vi "Input Registers Engine.vi"(10 "Parameters":variant, 11 "Process":refnum<class "Process.lvclass">) -> ()   [LabVIEW 2021, in "FPGA Addon Engine.lvlib"]
uses:
  FPGA Addon Engine.lvlib
  <vilib>/NI/NIVS Inline Async API/_VS Inline Async API/Process/Process.lvclass
  Types/Register Settings.ctl
  Addon Shared/Types/FPGA Addon Data Type.ctl
  Addon Shared/Types/Scalar Type.ctl
  <vilib>/NI/NIVS Inline Async API/_VS Inline Async API/Process/Process.lvclass/Process.ctl
  <vilib>/Platform/TimedLoop/XDataNode/timing_clust.ctl
  <vilib>/Platform/TimedLoop/XDataNode/nitl_modes.ctl
  <vilib>/Platform/TimedLoop/XDataNode/wakeup.ctl
  <vilib>/NI/NIVS Inline Async API/_Data Access Engine/Access Type Classes/Write/Write.lvclass/Write.ctl
  <vilib>/NI/NIVS Inline Async API/_Data Access Engine/Data Access Engine/Methods/Write.Data.vi
  <vilib>/NI/NIVS Inline Async API/_VS Inline Async API/Process/Data Member Access/Read Data Access.vi
  <vilib>/NI/NIVS Inline Async API/_VS Inline Async API/Error Handling Process/SubVIs/Error.ConvertArray.vi
  <vilib>/NI/NIVS Inline Async API/_Data Access Engine/Access Type Classes/Write/Write.ProcessData.vi
  <vilib>/NI/NIVS Inline Async API/_Data Access Engine/Access Type Classes/Write/Write.Buffer.vi
  <vilib>/NI/NIVS Inline Async API/_Data Access Engine/Access Type Classes/Write/Write.Commit.vi
  Addon Shared/SubVIs/Constants.vi
  <vilib>/NI/NIVS Inline Async API/_Data Access Engine/Data Access Engine/Methods/Write.Lookup.vi
  <vilib>/NI/NIVS Inline Async API/_Data Access Engine/Data Access Engine/Data Access Engine.lvclass
  <vilib>/platform/TimedLoop/XDataNode/XDataNode.xnode
  Addon Shared/FPGA Addon Shared.lvlib
  <vilib>/Platform/TimedLoop/XDataNode/XDNodeRunTimeDep.lvlib
panel:
  out "error out":errorcluster
  in  "error in (no error)":errorcluster
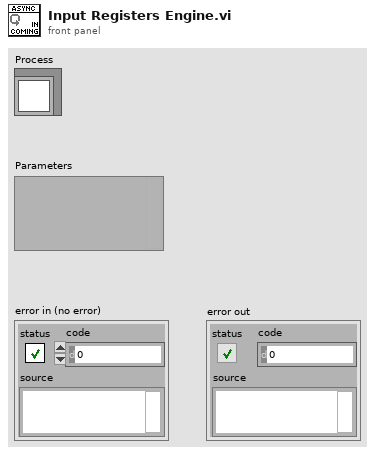
[diagram p1: front panel]
types:
  T1 = typedef "FPGA Addon Engine.lvlib/Register Settings.ctl" = cluster{"Name":string, "Data Type":T2, "session":u32, "Scalar Type":T3, "Index":i32, "Length":i32, "attributes":variant, "default value":variant}
  T2 = typedef "FPGA Addon Shared.lvlib/FPGA Addon Data Type.ctl" = enum8{"<Null>", "I8", "I16", "I32", "I64", "U8", "U16", "U32", "U64", "SGL", "Boolean", "Analog PWM In Settings", "Analog PWM In", "Digital PWM In Settings", "Digital PWM In", "Digital PWM Out", "Sine Out", "FXP", "FXP+/-24.5", "FXP+/-16.5", "FXP+/-32.8", "FXP+/-64.32", "FXP+/-16.7", "FXP+/-20.5", "FXP+/-27.5", "FXP+/-32.16", "FXP+16.3", "FXP+18.3", "Digital Static In", "Digital Static Out", "Digital Static In Settings", "Digital WSS Out", "Quad Encoder Settings", "Quad Encoder In", "Group"}
  T3 = typedef "FPGA Addon Shared.lvlib/Scalar Type.ctl" = enum16{"Standard", "Bitpacked"}
  T4 = typedef "Data Access Engine.lvlib/Data Access Engine.lvclass/Write.DVR.ctl" = refnum<data-value>
  T5 = typedef "XDNodeRunTimeDep.lvlib/timing_clust.ctl" = cluster{"Expected End [f-1]":u64, "Actual End [f-1]":u64, "Finished Late? [f-1]":bool, "Expected End [i-1]":u64, "Actual End [i-1]":u64, "Finished Late? [i-1]":bool, "Expected Start [i]":u64, "Actual Start [i]":u64, "Expected Start [f]":u64, "Actual Start [f]":u64, "Source Name":string, "Structure Name":string, "Period":i64, "Deadline":i64, "Offset":i64, "Start":i64, "Priority":i32, "Timeout":i32, "Mode":T6, "Wakeup Reason":T7, "Error":errorcluster, "Source Type":string, "Secondary Source Type":string, "Global End Time":u64, "Global Start Time":u64, "Frame Duration":u64, "Iteration Duration":u64, "Assigned CPU":i32, "I/O Scan Engine Mode":u32}
  T6 = typedef "XDNodeRunTimeDep.lvlib/nitl_modes.ctl" = enum32{"No Change", "Process missed periods, maintain original phase", "Discard missed periods, maintain original phase", "Process missed periods, ignore original phase", "Discard missed periods, ignore original phase"}
  T7 = typedef "XDNodeRunTimeDep.lvlib/wakeup.ctl" = enum32{"Normal", "Aborted", "Asynchronous wakeup", "Timing source error", "Timed loop error", "Timeout"}
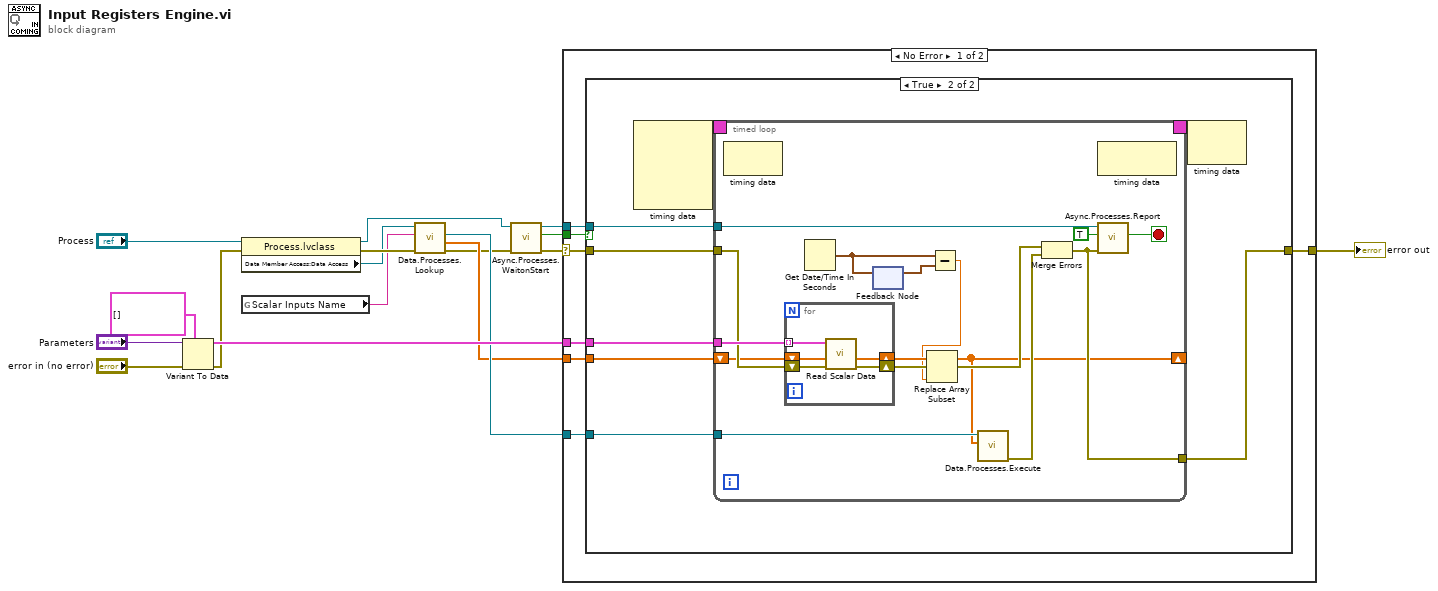
[diagram p0: block diagram]
diagram:
  n1 = Variant To Data(error in="error in (no error)", type=T1[] [] ("Parameters"), Variant="Parameters") -> (data=w11:T1[], error out=w3:errorcluster)
  n2 = property class="Process.lvclass"(reference="Process", error in=w3) -> (reference out=w7:refnum<class "Process.lvclass">, error out=w10:errorcluster, "Data Member Access:Data Access"=w9:refnum<class "Data Access Engine.lvclass">)
  n3 = global read "Constants.vi" "Scalar Inputs Name"() -> (w1:string)
  n4 = call-poly <vilib>:"Data.Processes.Lookup.vi"("error in (no error)"=w10, "Name"=w1, "Data Access API in"=w9) -> ("error out"=w4:errorcluster, "Initial Values"=w5:dbl[], "Ref"=w6:T4)  [unwired: 5 in, 1 out]
  n5 = call <vilib>:"Async.Processes.WaitonStart.vi"("error in (no error)"=w4, "Process"=w7) -> ("error out"=w15:errorcluster, "Execute"=w17:bool, "Process out"=w16:refnum<class "Process.lvclass">)  [unwired: 7 in]
  n6 = case shown="No Error" w15 {
    selector: w15 -> [w22 w58]
    tunnel: w17 -> [w24 _]
    tunnel: w16 -> [w23 _]
    tunnel: w11 -> [w21 _]
    tunnel: w6 -> [w20 _]
    tunnel: w5 -> [w19 _]
    tunnel: [w18 w58] -> w2
    frame No Error {
      n7 = case shown="True" w24 {
        tunnel: w23 -> [_ w33]
        tunnel: w22 -> [w25 w28]
        tunnel: w21 -> [_ w32]
        tunnel: w20 -> [_ w31]
        tunnel: w19 -> [_ w30]
        tunnel: [w25 w29] -> w18
        frame False {
        }
        frame True {
          n8 = node-c288() -> (w27:T5)  [unwired: 4 in]
          n9 = timed-loop {
            tunnel: w33 -> [w48]
            tunnel: w28 -> [w45]
            tunnel: w32 -> [w46]
            tunnel: w31 -> [w44]
            tunnel: [w41] -> w29
            shift-right: [w37] -> _
            shift-left: w30 -> [w40]
            timing: w27 -> [_]
            timing-out: [_] -> w26
            stop <- w47 stop-if-true
            n10 = node-c288() -> ()  [unwired: 1 in, 1 out]
            n11 = for {
              shift-right: [w52] -> w39
              shift-left: w40 -> [w53]
              shift-right: [w54] -> w42
              shift-left: w45 -> [w55]
              tunnel: w46 -> [w51] mode=indexing
              n12 = call "Read Scalar Data.vi"("error in (no error)"=w55, "Values"=w53, "Cluster"=w51) -> ("error out"=w54:errorcluster, "Values"=w52:dbl[])  [unwired: 7 in]
            }
            n13 = Get Date/Time In Seconds() -> (seconds since 1Jan1904=w35:timestamp)
            n14 = feedback-in #1(w35) -> ()
            n15 = feedback #1() -> (w36:timestamp)  [unwired: 1 in]
            n16 = Subtract(x=w35, y=w36) -> (x-y=w34:dbl)
            n17 = Replace Array Subset(array=w39, new element=w34) -> (w37:dbl[])  [unwired: 1 in]
            n18 = call-poly <vilib>:"Data.Processes.Execute.vi"("Values"=w37, "Ref"=w44) -> ("error out"=w43:errorcluster)  [unwired: 9 in]
            n19 = Merge Errors(w42, w43) -> (w41:errorcluster)
            n20 = node-c288() -> ()  [unwired: 1 in, 1 out]
            n21 = call <vilib>:"Async.Processes.Report.vi"("Error"=w41, "Stop Async on Error?"=TRUE, "Process in"=w48) -> ("Stop"=w47:bool)  [unwired: 7 in, 1 out]
          }
          n22 = node-c288(w26) -> ()  [unwired: 1 out]
        }
      }
    }
    frame Error {
    }
  }
  "error out" <- w2
